vi "Create Code String.vi"   [LabVIEW 2016, in "Code String.lvclass"]
uses:
  Code String.lvclass
  Code String LV/Code String LV.lvclass
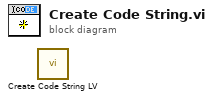
[diagram p0: block diagram]
diagram:
  n1 = call "Create Code String LV.vi"() -> ()  [unwired: 14 in, 2 out]
